vi "LDO Line Transient v2 - Flat.vi"(11 "error in (no error)":errorcluster) -> (15 "error out":errorcluster)   [LabVIEW 2020]
uses:
  <instrlib>/niScope/Controls/niScope vertical coupling.ctl
  <instrlib>/niScope/Controls/niScope trigger source digital.ctl
  <instrlib>/niDCPower/nidcpower.llb/niDCPower Aperture Time Units.ctl
  <instrlib>/niDCPower/nidcpower.llb/niDCPower Source Mode.ctl
  <instrlib>/niDCPower/nidcpower.llb/niDCPower Output Function.ctl
  <instrlib>/niDCPower/nidcpower.llb/niDCPower Export Signal - Signal.ctl
  <instrlib>/niDCPower/nidcpower.llb/niDCPower Wait For Event - Event.ctl
  <instrlib>/niScope/Controls/niScope trigger slope.ctl
  <instrlib>/niScope/Configure/Trigger/niScope Configure Trigger Digital.vi
  <instrlib>/niScope/Acquire/Fetch/niScope Multi Fetch Cluster.vi
  <instrlib>/niScope/Utility/niScope Get Channel Name From String.vi
  <vilib>/gmath/NI_Gmath.lvlib
  LDO Line Transient.lvlib
  <vilib>/gmath/NumericalOptimization/Nonlinear Curve Fit LM formula string.vi
panel:
  out "Horizontal:Number of Records":i32=400000
  out "Horizontal:Min Sample Rate":dbl=1000000.0
  out "Measurement:Measure Record Length":i32=10
  out "Measurement:Aperture Time":dbl=4.9999999999999996e-06
  out "Source:Advanced:Source Delay":dbl=3.086419753086419e-08
  in  "Tab Control":T1(tab)=enum."Waveform"
  in  "Scope":refnum<k15>="PXI1Slot5"
  in  "Load SMU":refnum<k15>="SMU1"
  in  "Source SMU":refnum<k15>="SMU1"
  in  "Load SMU Voltage Limit (V)":dbl=8.0
  in  "Load SMU Voltage Limit Range (V)":dbl=8.0
  in  "Load SMU Current Level Range (A)":dbl=3.0
  in  "Load SMU Channel":string="1"
  in  "Load Current (A)":dbl=-0.05
  in  "Min. Record Length":i32=400000
  in  "Min. Sampling Rate":dbl=1000000.0
  in  "Trigger Modifier":i32(ring) items=["None", "Auto"]
  in  "Reference Position":dbl
  in  "Input Impedance":u32(ring) items=["1 Mega Ohm"=0, "50 Ohm"=2]
  in  "Trigger Delay (sec)":dbl
  in  "Max. Input Frequency (Hz)":dbl
  in  "Vertical Offset (V)":dbl
  in  "Probe Attentuation":dbl=1.0
  in  "Vertical Range (V)":dbl=5.0
  in  "Scope Channel":string="0,1"
  in  "Source SMU Current Limit (A)":dbl=0.2
  in  "Source SMU Transient Response":i32(ring)=1039 items=["Slow"=1041, "Normal"=1038, "Fast"=1039, "Custom"=1042]
  in  "Source SMU Record Length":i32=10
  in  "Source SMU Aperture Time (sec)":dbl=5e-06
  in  "Source SMU Current Limit Range (A)":dbl=0.2
  in  "Source SMU Voltage Level Range (V)":dbl=8.0
  in  "Source SMU Channel":string="0"
  in  "Source  SMU Steady State Voltage (V)":dbl=4.0
  in  "Vertical Coupling":T2 items=["AC", "DC", "Ground"]
  in  "Trigger Source":T3="VAL_PFI_0" caption="trigger source (RTSI 0)"
  in  "Recovery Level (V)":dbl=0.1
  in  "Vin2 Voltage Level Width (sec)":dbl=0.1
  in  "Source Voltage 2 - Vin2":dbl=5.0
  in  "Source Voltage 1 - Vin1":dbl=4.0
  out "Settling time (ms)":dbl=0.008841
  out "Mixed Signal Graph":cluster{waveform(dbl), waveform(dbl)}(graph)={{"t0"=timestamp(0 s since 1904-01-01), "dt"=4.9999999999999996e-06, "Y"=array[40000 elements]}, {"t0"=timestamp(0 s since 1904-01-01), "dt"=4.9999999999999996e-06, "Y"=array[40000 elements]}}
  out "Waveform(s)":T4(graph) caption="Instantaneous Load Transient Waveform"
  out "XY Graph 2":cluster{dbl[], dbl[]}[](graph)
  out "XY Graph":cluster{dbl[], "wfm":dbl[]}[](graph)
  # "Line Transient Measurement - Flat VI"
  # "Source SMU Config"
  # "Scope Config"
  # "Load SMU Config"
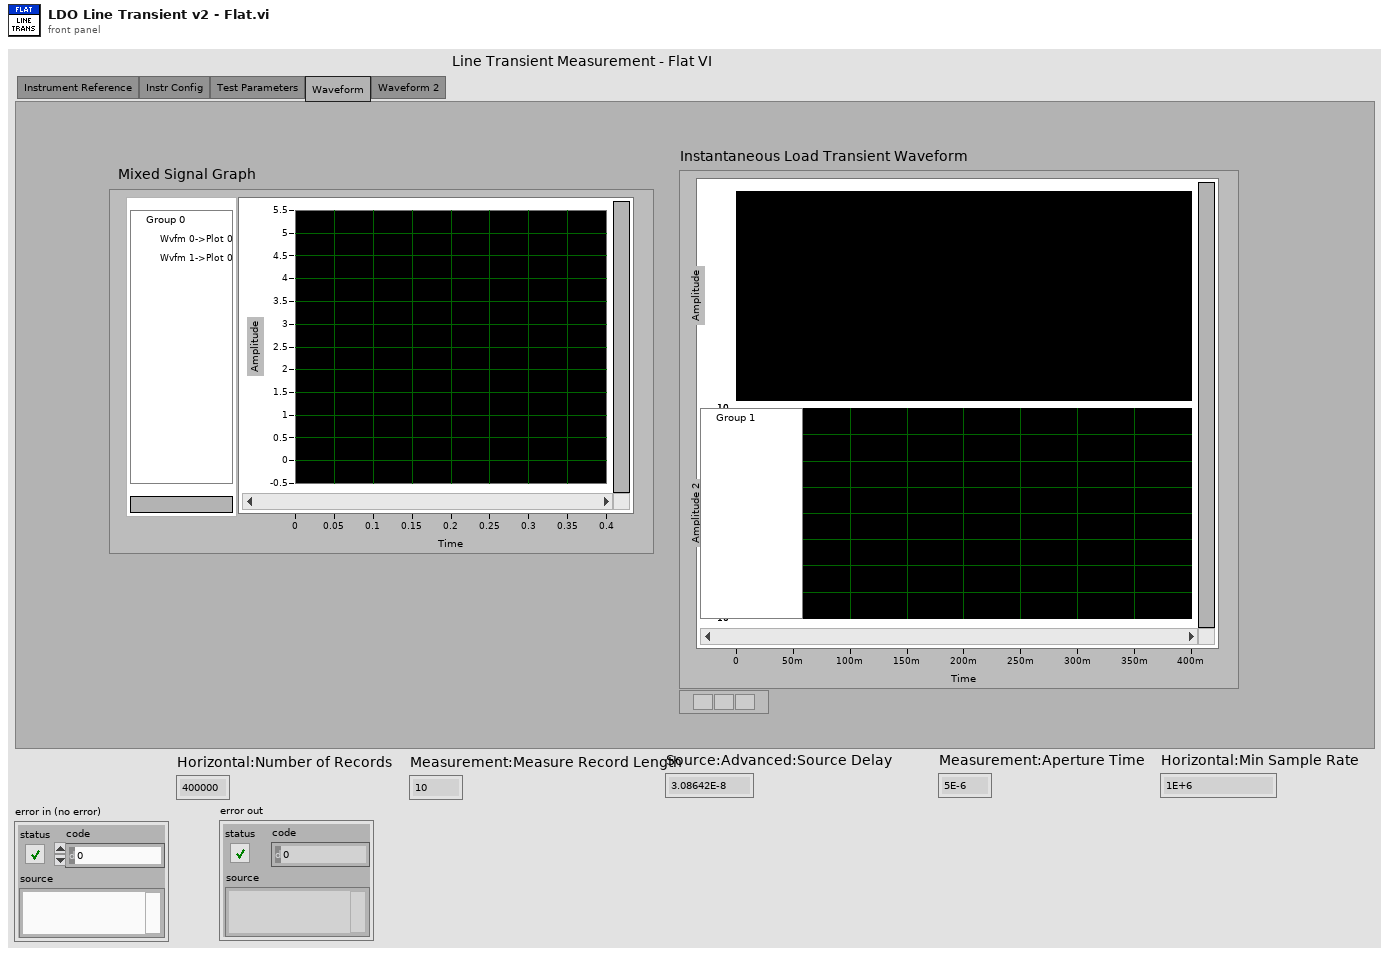
[diagram p1: front panel]
types:
  T1 = enum32{"Instrument Reference", "Instr Config", "Test Parameters", "Waveform", "Waveform 2"}
  T2 = typedef "niScope vertical coupling.ctl" = i32
  T3 = typedef "niScope trigger source digital.ctl" = string
  T4 = cluster{"relativeInitialX":dbl, "xIncrement":dbl, "wfm":dbl[]}[]
  T5 = typedef "niDCPower Output Function.ctl" = i32
  T6 = typedef "niDCPower Source Mode.ctl" = i32
  T7 = typedef "niScope trigger slope.ctl" = i32
  T8 = typedef "niDCPower Wait For Event - Event.ctl" = i32
  T9 = typedef "niDCPower Export Signal - Signal.ctl" = i32
  T10 = typedef "niDCPower Aperture Time Units.ctl" = i32
  T11 = cluster{"relativeInitialX":dbl, "xIncrement":dbl, "wfm":dbl[]}
  T12 = cluster{"model":string, "Parameters":string[], "x":string}
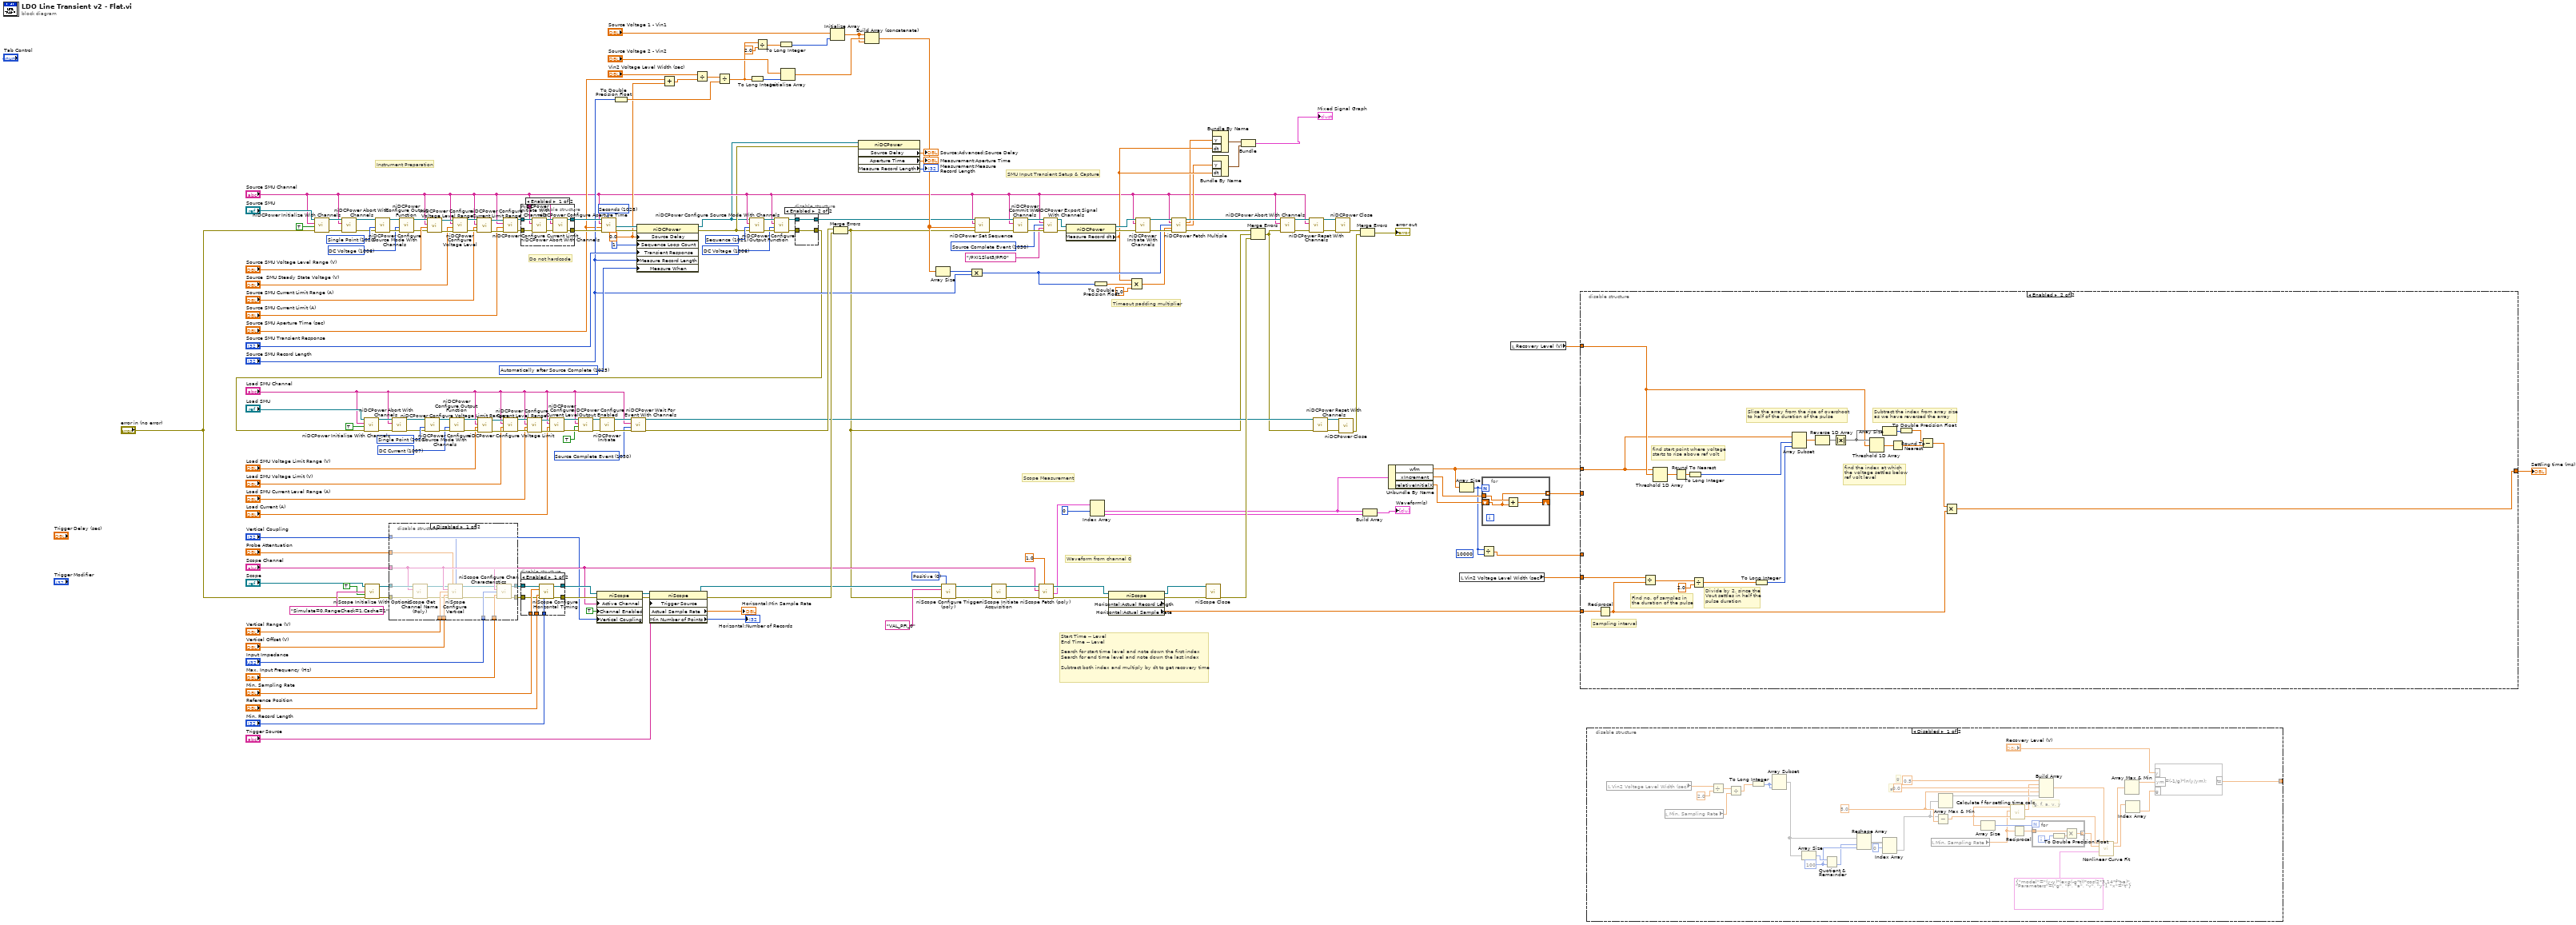
[diagram p0: block diagram]
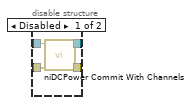
[diagram p4: hidden frame]
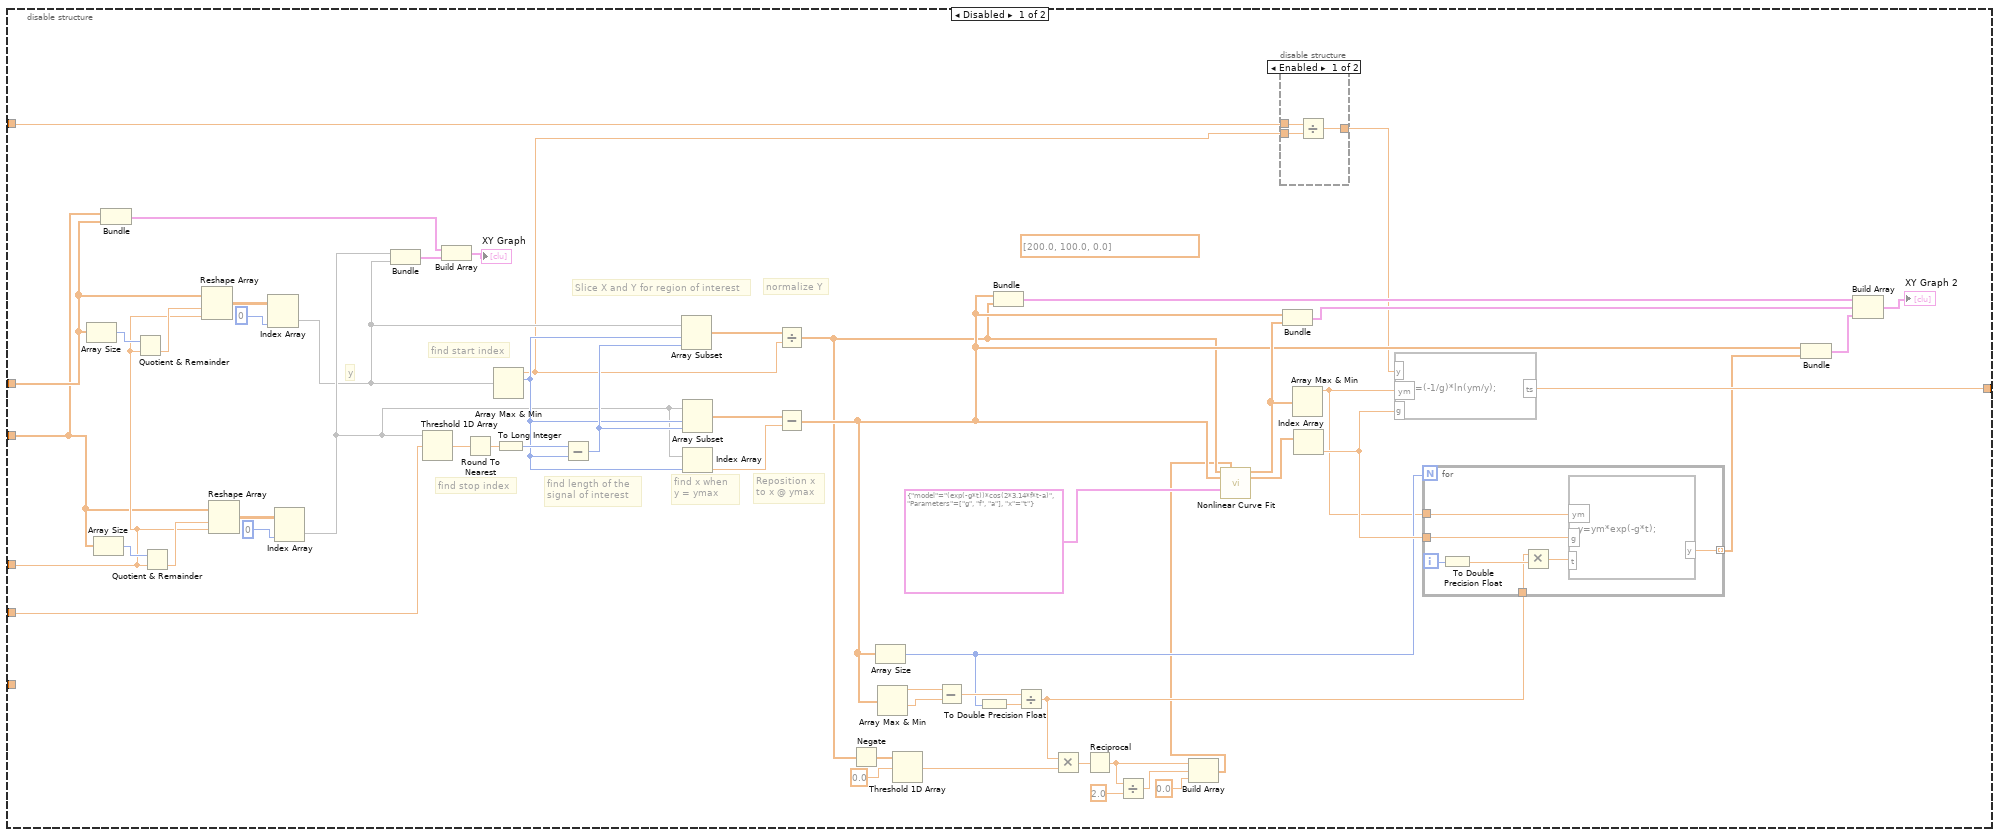
[diagram p5: hidden frame]
diagram:
  (unwired) 10000 ("y")
  w57 = T5 1006 items=["DC Voltage"=1006, "DC Current"=1007, "Pulse Voltage"=1049, "Pulse Current"=1050] ("output function")
  w58 = T6 1021 items=["Single Point"=1020, "Sequence"=1021] ("source mode")
  w51 = T7 0 items=["Positive", "Negative"] ("trigger slope")
  w80 = T8 1030 items=["Source Complete Event"=1030, "Measure Complete Event"=1031, "Sequence Iteration Complete Event"=1032, "Sequence Engine Done Event"=1033, "Pulse Complete Event"=1051, "Ready For Pulse Trigger Event"=1052] ("event")
  w113 = T9 1030 items=["Source Complete Event"=1030, "Measure Complete Event"=1031, "Sequence Iteration Complete Event"=1032, "Sequence Engine Done Event"=1033, "Pulse Complete Event"=1051, "Ready For Pulse Trigger Event"=1052, "Start Trigger"=1034, "Source Trigger"=1035, "Measure Trigger"=1036, "Sequence Advance Trigger"=1037, "Pulse Trigger"=1053] ("signal")
  w153 = T5 1007 items=["DC Voltage"=1006, "DC Current"=1007, "Pulse Voltage"=1049, "Pulse Current"=1050] ("output function")
  w154 = T6 1020 items=["Single Point"=1020, "Sequence"=1021] ("source mode")
  w162 = 1025 items=["Automatically after Source Complete"=1025, "On Demand"=1026, "On Measure Trigger"=1027] ("Measurement:Advanced:Measure When")
  w42 = 0.0 ("Source:Advanced:Source Delay")
  w169 = T10 1028 items=["Seconds"=1028, "Powerline Cycles"=1029] ("aperture time units")
  w172 = T5 1006 items=["DC Voltage"=1006, "DC Current"=1007, "Pulse Voltage"=1049, "Pulse Current"=1050] ("output function")
  w173 = T6 1020 items=["Single Point"=1020, "Sequence"=1021] ("source mode")
  # "Do not hardcode"
  # "Start Time -- Level\nEnd Time -- Level\n\nSearch for start time level and note down the first index\nSearch for end time level and note down the last index\n\nSubtract both index and multiply by dt to get recovery time"
  # "SMU Input Transient Setup & Capture"
  # "Scope Measurement"
  # "Waveform from channel 0"
  # "Timeout padding multiplier"
  # "Instrument Preparation"
  n1 = call <instrlib>:"niDCPower Initialize With Channels.vi"("error in (no error)"="error in (no error)", "reset (false)"=TRUE, "channels"="Source SMU Channel", "resource name"="Source SMU") -> ("error out"=w168:errorcluster, "instrument handle out"=w166:refnum<k15>)  [unwired: 1 in, 5 out]
  n2 = call <instrlib>:"niDCPower Abort With Channels.vi"("error in (no error)"=w168, "channel name"="Source SMU Channel", "instrument handle"=w166) -> ("error out"=w167:errorcluster, "instrument handle out"=w165:refnum<k15>)  [unwired: 7 in]
  n3 = call <instrlib>:"niScope Initialize With Options.vi"("resource name"="Scope", "option string"="Simulate=0,RangeCheck=1,Cache=1", "reset device"=TRUE, "error in"="error in (no error)") -> ("instrument handle"=w139:refnum<k15>, "error out"=w138:errorcluster)  [unwired: 10 in]
  n4 = call <instrlib>:"niDCPower Configure Source Mode With Channels.vi"("error in (no error)"=w167, "source mode"=w173, "instrument handle"=w165) -> ("error out"=w174:errorcluster, "instrument handle out"=w175:refnum<k15>)  [unwired: 7 in]
  n5 = disable-structure shown="Disabled" {
    disable-tunnel: w139 -> [w202 w203]
    disable-tunnel: w138 -> [w201 w204]
    disable-tunnel: "Probe Attentuation" -> [w200 _]
    disable-tunnel: "Vertical Range (V)" -> [w199 _]
    disable-tunnel: "Vertical Offset (V)" -> [w198 _]
    disable-tunnel: "Max. Input Frequency (Hz)" -> [w197 _]
    disable-tunnel: "Input Impedance" -> [w196 _]
    disable-tunnel: "Scope Channel" -> [w195 _]
    disable-tunnel: "Vertical Coupling" -> [w194 _]
    disable-tunnel: [w189 w204] -> w12
    disable-tunnel: [w188 w203] -> w11
    frame Disabled {
      n6 = call-poly <instrlib>:"niScope Get Channel Name (Poly).vi"("instrument handle"=w202, "index"=w195, "error in"=w201) -> ("instrument handle out"=w193:refnum<k15>, "error out"=w192:errorcluster)  [unwired: 10 in, 1 out]
      n7 = call <instrlib>:"niScope Configure Vertical.vi"("instrument handle"=w193, "probe attenuation"=w200, "vertical coupling"=w194, "channels"=w195, "vertical range"=w199, "vertical offset"=w198, "error in"=w192) -> ("instrument handle out"=w191:refnum<k15>, "error out"=w190:errorcluster)  [unwired: 7 in]
      n8 = call <instrlib>:"niScope Configure Chan Characteristics.vi"("instrument handle"=w191, "channels"=w195, "input impedance"=w196, "maximum input frequency"=w197, "error in"=w190) -> ("instrument handle out"=w188:refnum<k15>, "error out"=w189:errorcluster)  [unwired: 9 in]
    }
    frame Enabled {
    }
  }
  n9 = call <instrlib>:"niDCPower Configure Output Function.vi"("error in (no error)"=w174, "output function"=w172, "instrument handle"=w175) -> ("error out"=w170:errorcluster, "instrument handle out"=w171:refnum<k15>)  [unwired: 7 in]
  n10 = call <instrlib>:"niDCPower Configure Voltage Level Range.vi"("error in (no error)"=w170, "voltage level range"="Source SMU Voltage Level Range (V)", "channel name"="Source SMU Channel", "instrument handle"=w171) -> ("error out"=w187:errorcluster, "instrument handle out"=w186:refnum<k15>)  [unwired: 6 in]
  n11 = call <instrlib>:"niDCPower Configure Voltage Level.vi"("error in (no error)"=w187, "voltage level"="Source  SMU Steady State Voltage (V)", "channel name"="Source SMU Channel", "instrument handle"=w186) -> ("error out"=w185:errorcluster, "instrument handle out"=w184:refnum<k15>)  [unwired: 6 in]
  n12 = call <instrlib>:"niDCPower Configure Current Limit Range.vi"("error in (no error)"=w185, "current limit range"="Source SMU Current Limit Range (A)", "channel name"="Source SMU Channel", "instrument handle"=w184) -> ("error out"=w183:errorcluster, "instrument handle out"=w182:refnum<k15>)  [unwired: 6 in]
  n13 = call <instrlib>:"niDCPower Configure Current Limit.vi"("error in (no error)"=w183, "current limit"="Source SMU Current Limit (A)", "channel name"="Source SMU Channel", "instrument handle"=w182) -> ("error out"=w55:errorcluster, "instrument handle out"=w53:refnum<k15>)  [unwired: 6 in]
  n14 = disable-structure shown="Enabled" {
    disable-tunnel: w55 -> [w209 w212]
    disable-tunnel: [w208 w212] -> w54
    disable-tunnel: w53 -> [w207 w213]
    disable-tunnel: [w206 w213] -> w52
    disable-tunnel: "Source SMU Channel" -> [w205 _]
    frame Enabled {
      n15 = call <instrlib>:"niDCPower Initiate With Channels.vi"("error in (no error)"=w209, "channel name"=w205, "instrument handle"=w207) -> ("error out"=w211:errorcluster, "instrument handle out"=w210:refnum<k15>)  [unwired: 7 in]
      n16 = call <instrlib>:"niDCPower Abort With Channels.vi"("error in (no error)"=w211, "channel name"=w205, "instrument handle"=w210) -> ("error out"=w208:errorcluster, "instrument handle out"=w206:refnum<k15>)  [unwired: 7 in]
    }
    frame Disabled {
    }
  }
  n17 = disable-structure shown="Enabled" {
    disable-tunnel: "Min. Record Length" -> [w220 _]
    disable-tunnel: "Reference Position" -> [w219 _]
    disable-tunnel: "Min. Sampling Rate" -> [w218 _]
    disable-tunnel: [w217 w221] -> w21
    disable-tunnel: [w216 w222] -> w19
    disable-tunnel: w12 -> [w215 w221]
    disable-tunnel: w11 -> [w214 w222]
    frame Enabled {
      n18 = call <instrlib>:"niScope Configure Horizontal Timing.vi"("instrument handle"=w214, "min sample rate"=w218, "reference position"=w219, "error in"=w215, "min record length"=w220) -> ("instrument handle out"=w216:refnum<k15>, "error out"=w217:errorcluster)  [unwired: 9 in]
    }
    frame Disabled {
    }
  }
  n19 = property class="niScope"(reference=w19, error in=w21, "Active Channel"="Scope Channel", "Channel Enabled"=TRUE ("Vertical:Channel Enabled"), "Vertical Coupling"="Vertical Coupling") -> (reference out=w18:refnum<k15>, error out=w20:errorcluster)
  n20 = call <instrlib>:"niDCPower Configure Aperture Time.vi"("aperture time units"=w169, "error in (no error)"=w54, "aperture time"="Source SMU Aperture Time (sec)", "channel name"="Source SMU Channel", "instrument handle"=w52) -> ("error out"=w88:errorcluster, "instrument handle out"=w49:refnum<k15>)  [unwired: 5 out]
  n21 = To Double Precision Float(number="Source SMU Record Length") -> (double precision float=w46:dbl)
  n22 = property class="niDCPower"(reference=w49, error in=w88, "Source Delay"=w42, "Sequence Loop Count"=1 ("Source:Advanced:Sequence Loop Count"), "Transient Response"="Source SMU Transient Response", "Measure Record Length"="Source SMU Record Length", "Measure When"=w162) -> (reference out=w22:refnum<k15>, error out=w23:errorcluster)
  n23 = property class="niScope"(reference=w18, error in=w20, "Trigger Source"="Trigger Source") -> (reference out=w75:refnum<k15>, error out=w77:errorcluster, "Actual Sample Rate"=→"Horizontal:Min Sample Rate":dbl, "Min Number of Points"=→"Horizontal:Number of Records":i32)
  n24 = Add(x="Source SMU Aperture Time (sec)", y=w42) -> (x+y=w43:dbl)
  n25 = Divide(x="Vin2 Voltage Level Width (sec)", y=w43) -> (x/y=w48:dbl)
  n26 = Divide(x=w48, y=w46) -> (x/y=w45:dbl)
  n27 = call <instrlib>:"niDCPower Configure Source Mode With Channels.vi"("error in (no error)"=w23, "source mode"=w58, "channel name"="Source SMU Channel", "instrument handle"=w22) -> ("error out"=w59:errorcluster, "instrument handle out"=w56:refnum<k15>)  [unwired: 6 in]
  n28 = To Long Integer(number=w45) -> (32bit integer=w125:i32)
  n29 = Divide(x=w45, y=2.0) -> (x/y=w121:dbl)
  n30 = call <instrlib>:"niDCPower Configure Output Function.vi"("error in (no error)"=w59, "output function"=w57, "channel name"="Source SMU Channel", "instrument handle"=w56) -> ("error out"=w27:errorcluster, "instrument handle out"=w26:refnum<k15>)  [unwired: 6 in]
  n31 = To Long Integer(number=w121) -> (32bit integer=w120:i32)
  n32 = Initialize Array("Source Voltage 2 - Vin2", w125) -> (w119:dbl[])
  n33 = disable-structure shown="Enabled" {
    disable-tunnel: w27 -> [w226 w227]
    disable-tunnel: [w225 w227] -> w9
    disable-tunnel: w26 -> [w224 w228]
    disable-tunnel: [w223 w228] -> w25
    frame Disabled {
      n34 = call <instrlib>:"niDCPower Commit With Channels.vi"("error in (no error)"=w226, "instrument handle"=w224) -> ("error out"=w225:errorcluster, "instrument handle out"=w223:refnum<k15>)  [unwired: 8 in]
    }
    frame Enabled {
    }
  }
  n35 = call <instrlib>:"niDCPower Initialize With Channels.vi"("error in (no error)"=w9, "reset (false)"=TRUE, "channels"="Load SMU Channel", "resource name"="Load SMU") -> ("error out"=w150:errorcluster, "instrument handle out"=w148:refnum<k15>)  [unwired: 1 in, 5 out]
  n36 = call <instrlib>:"niDCPower Abort With Channels.vi"("error in (no error)"=w150, "channel name"="Load SMU Channel", "instrument handle"=w148) -> ("error out"=w149:errorcluster, "instrument handle out"=w147:refnum<k15>)  [unwired: 7 in]
  n37 = call <instrlib>:"niDCPower Configure Source Mode With Channels.vi"("error in (no error)"=w149, "source mode"=w154, "instrument handle"=w147) -> ("error out"=w155:errorcluster, "instrument handle out"=w156:refnum<k15>)  [unwired: 7 in]
  n38 = call <instrlib>:"niDCPower Configure Output Function.vi"("error in (no error)"=w155, "output function"=w153, "instrument handle"=w156) -> ("error out"=w151:errorcluster, "instrument handle out"=w152:refnum<k15>)  [unwired: 7 in]
  n39 = call <instrlib>:"niDCPower Configure Voltage Limit Range.vi"("error in (no error)"=w151, "voltage limit range"="Load SMU Voltage Limit Range (V)", "channel name"="Load SMU Channel", "instrument handle"=w152) -> ("error out"=w161:errorcluster, "instrument handle out"=w160:refnum<k15>)  [unwired: 6 in]
  n40 = call <instrlib>:"niDCPower Configure Voltage Limit.vi"("error in (no error)"=w161, "voltage limit"="Load SMU Voltage Limit (V)", "channel name"="Load SMU Channel", "instrument handle"=w160) -> ("error out"=w159:errorcluster, "instrument handle out"=w158:refnum<k15>)  [unwired: 6 in]
  n41 = call <instrlib>:"niDCPower Configure Current Level Range.vi"("error in (no error)"=w159, "current level range"="Load SMU Current Level Range (A)", "channel name"="Load SMU Channel", "instrument handle"=w158) -> ("error out"=w144:errorcluster, "instrument handle out"=w145:refnum<k15>)  [unwired: 6 in]
  n42 = call <instrlib>:"niDCPower Configure Current Level.vi"("error in (no error)"=w144, "current level"="Load Current (A)", "channel name"="Load SMU Channel", "instrument handle"=w145) -> ("error out"=w85:errorcluster, "instrument handle out"=w82:refnum<k15>)  [unwired: 6 in]
  n43 = call <instrlib>:"niDCPower Configure Output Enabled.vi"("error in (no error)"=w85, "output enabled"=TRUE, "channel name"="Load SMU Channel", "instrument handle"=w82) -> ("error out"=w84:errorcluster, "instrument handle out"=w87:refnum<k15>)  [unwired: 6 in]
  n44 = call <instrlib>:"niDCPower Initiate.vi"("error in (no error)"=w84, "instrument handle"=w87) -> ("error out"=w83:errorcluster, "instrument handle out"=w86:refnum<k15>)  [unwired: 8 in]
  n45 = call <instrlib>:"niDCPower Wait For Event With Channels.vi"("error in (no error)"=w83, "event"=w80, "channel name"="Load SMU Channel", "instrument handle"=w86) -> ("error out"=w78:errorcluster, "instrument handle out"=w63:refnum<k15>)  [unwired: 6 in]
  n46 = Initialize Array("Source Voltage 1 - Vin1", w120) -> (w118:dbl[])
  n47 = Merge Errors(w78, w77) -> (w7:errorcluster)
  n48 = property class="niDCPower"(reference=w22, error in=w23) -> ("Source Delay"=→"Source:Advanced:Source Delay":dbl, "Aperture Time"=→"Measurement:Aperture Time":dbl, "Measure Record Length"=→"Measurement:Measure Record Length":i32)  [unwired: 2 out]
  n49 = Build Array (concatenate)(w118, w119, w118) -> (w109:dbl[])
  n50 = Array Size(array=w109) -> (size(s)=w108:i32)
  n51 = call-poly <instrlib>:"niScope Configure Trigger (poly).vi"("instrument handle"=w75, "trigger slope"=w51, "trigger source"=T3 "VAL_PFI_0", "error in"=w7) -> ("instrument handle out"=w76:refnum<k15>, "error out"=w90:errorcluster)  [unwired: 10 in]
  n52 = Compound Arithmetic op=MULTIPLY(w108, "Source SMU Record Length") -> (w101:i32)
  n53 = call <instrlib>:"niDCPower Set Sequence.vi"("error in (no error)"=w7, "values"=w109, "channel name"="Source SMU Channel", "instrument handle"=w25) -> ("error out"=w117:errorcluster, "instrument handle out"=w116:refnum<k15>)  [unwired: 1 in, 5 out]
  n54 = call <instrlib>:"niScope Initiate Acquisition.vi"("instrument handle"=w76, "error in"=w90) -> ("instrument handle out"=w73:refnum<k15>, "error out"=w89:errorcluster)  [unwired: 12 in]
  n55 = call <instrlib>:"niDCPower Commit With Channels.vi"("error in (no error)"=w117, "channel name"="Source SMU Channel", "instrument handle"=w116) -> ("error out"=w115:errorcluster, "instrument handle out"=w114:refnum<k15>)  [unwired: 7 in]
  n56 = call-poly <instrlib>:"niScope Fetch (poly).vi"("timeout"=1.0, "error in"=w89, "channels"="Scope Channel", "instrument handle"=w73) -> ("error out"=w91:errorcluster, "waveform"=w70:T4, "instrument handle out"=w71:refnum<k15>)  [unwired: 4 in, 1 out]
  n57 = call <instrlib>:"niDCPower Export Signal With Channels.vi"("instrument handle"=w114, "channel name"="Source SMU Channel", "signal"=w113, "output terminal"=tag "/PXI1Slot5/PFI0", "error in (no error)"=w115) -> ("instrument handle out"=w110:refnum<k15>, "error out"=w111:errorcluster)  [unwired: 9 in]
  n58 = property class="niDCPower"(reference=w110, error in=w111) -> (reference out=w104:refnum<k15>, error out=w105:errorcluster, "Measure Record dt"=w94:dbl)
  n59 = Index Array(array=w70, index #1=0 ("index")) -> (element #1=w41:T11, element #2=w1:T11)  [unwired: 1 in]
  n60 = To Double Precision Float(number=w101) -> (double precision float=w106:dbl)
  n61 = property class="niScope" props=["Horizontal:Actual Record Length", "Horizontal:Actual Sample Rate"](reference=w71, error in=w91) -> (reference out=w67:refnum<k15>, error out=w68:errorcluster, "Horizontal:Actual Sample Rate"=w31:dbl)  [unwired: 1 out]
  n62 = Compound Arithmetic op=MULTIPLY(w94, w106, 2.0 ("value")) -> (w100:dbl)
  n63 = call <instrlib>:"niDCPower Initiate With Channels.vi"("error in (no error)"=w105, "channel name"="Source SMU Channel", "instrument handle"=w104) -> ("error out"=w103:errorcluster, "instrument handle out"=w102:refnum<k15>)  [unwired: 7 in]
  n64 = call <instrlib>:"niDCPower Fetch Multiple.vi"("instrument handle"=w102, "channel name"="Source SMU Channel", "count (1)"=w101, "timeout (sec)"=w100, "error in (no error)"=w103) -> ("instrument handle out"=w99:refnum<k15>, "voltage measurements"=w62:dbl[], "current measurements"=w93:dbl[], "error out"=w8:errorcluster)  [unwired: 7 out]
  n65 = call <instrlib>:"niScope Close.vi"("instrument handle"=w67, "error in"=w68) -> ("error out"=w66:errorcluster)  [unwired: 13 in]
  n66 = Bundle By Name("Y"=w62, "dt"=w94) -> (w92:waveform(dbl))  [unwired: 1 out]
  n67 = Bundle By Name("Y"=w93, "dt"=w94) -> (w61:waveform(dbl))  [unwired: 1 out]
  n68 = Bundle(w92, w61) -> (→"Mixed Signal Graph":cluster{waveform(dbl), waveform(dbl)})  [unwired: 1 in]
  n69 = Merge Errors(w8, w7, w66) -> (w6:errorcluster)
  n70 = call <instrlib>:"niDCPower Abort With Channels.vi"("error in (no error)"=w6, "channel name"="Source SMU Channel", "instrument handle"=w99) -> ("error out"=w97:errorcluster, "instrument handle out"=w95:refnum<k15>)  [unwired: 7 in]
  n71 = call <instrlib>:"niDCPower Reset With Channels.vi"("error in (no error)"=w97, "channel name"="Source SMU Channel", "instrument handle"=w95) -> ("error out"=w96:errorcluster, "instrument handle out"=w98:refnum<k15>)  [unwired: 7 in]
  n72 = call <instrlib>:"niDCPower Reset With Channels.vi"("error in (no error)"=w6, "instrument handle"=w63) -> ("error out"=w64:errorcluster, "instrument handle out"=w65:refnum<k15>)  [unwired: 8 in]
  n73 = call <instrlib>:"niDCPower Close.vi"("error in (no error)"=w96, "instrument handle"=w98) -> ("error out"=w5:errorcluster)  [unwired: 9 out]
  n74 = call <instrlib>:"niDCPower Close.vi"("error in (no error)"=w64, "instrument handle"=w65) -> ("error out"=w4:errorcluster)  [unwired: 9 out]
  n75 = Merge Errors(w5, w4) -> (→"error out":errorcluster)
  n76 = Build Array(w41, w1) -> (→"Waveform(s)":T4)
  n77 = Unbundle By Name(w41) -> ("wfm"=w36:dbl[], "xIncrement"=w39:dbl, "relativeInitialX"=w40:dbl)
  n78 = Array Size(array=w36) -> (size(s)=w34:i32)
  n79 = local read "Vin2 Voltage Level Width (sec)"() -> (w33:dbl)
  n80 = Divide(x=w34, y=w34) -> (x/y=w37:dbl)
  n81 = for {
    N: w34 -> [_]
    tunnel: w39 -> [w231]
    shift-right: [w230] -> _
    shift-left: w40 -> [w229]
    tunnel: [w229] -> w35 mode=indexing
    n82 = Add(x=w231, y=w229) -> (x+y=w230:dbl)
  }
  n83 = local read "Recovery Level (V)"() -> (w32:dbl)
  n84 = disable-structure shown="Enabled" {
    disable-tunnel: [w277 w303] -> w38
    disable-tunnel: w37 -> [w258 _]
    disable-tunnel: w36 -> [w241 w300]
    disable-tunnel: w35 -> [w240 _]
    disable-tunnel: w33 -> [w233 w299]
    disable-tunnel: w32 -> [w232 w301]
    disable-tunnel: w31 -> [_ w302]
    frame Disabled {
      (unwired) dbl[] [200.0, 100.0, 0.0] ("initial parameters")
      # "find x when \ny = ymax"
      # "Reposition x \nto x @ ymax"
      # "normalize Y"
      # "Slice X and Y for region of interest"
      # "find length of the \nsignal of interest"
      # "find stop index"
      # "find start index"
      # "y"
      n85 = Array Size(array=w241) -> (size(s)=w267:i32)
      n86 = Array Size(array=w240) -> (size(s)=w271:i32)
      n87 = Bundle(w240, "wfm"=w241) -> (w238:cluster{dbl[], "wfm":dbl[]})  [unwired: 1 in]
      n88 = Quotient & Remainder(x=w267, y=w258) -> (floor(x/y)=w266:dbl)  [unwired: 1 out]
      n89 = Quotient & Remainder(x=w271, y=w258) -> (floor(x/y)=w270:dbl)  [unwired: 1 out]
      n90 = Reshape Array(w241, w266, w258) -> (w265:dbl[][])
      n91 = Reshape Array(w240, w270, w258) -> (w269:dbl[][])
      n92 = Index Array(array=w265, index (col)=0 ("index (row)")) -> (element=w264:dbl[])  [unwired: 1 in]
      n93 = Index Array(array=w269, index (col)=0 ("index (row)")) -> (element=w268:dbl[])  [unwired: 1 in]
      n94 = Bundle(w268, "wfm"=w264) -> (w275:cluster{dbl[], "wfm":dbl[]})  [unwired: 1 in]
      n95 = Threshold 1D Array(2:w233, 3:w268) -> (0:w286:dbl)  [unwired: 1 in]
      n96 = Build Array(w238, w275) -> (→"XY Graph":cluster{dbl[], "wfm":dbl[]}[])
      n97 = Round To Nearest(number=w286) -> (nearest integer value=w287:dbl)
      n98 = Array Max & Min(array=w264) -> (max value=w236:dbl, max index (indices)=w281:i32)  [unwired: 2 out]
      n99 = To Long Integer(number=w287) -> (32bit integer=w285:i32)
      n100 = Subtract(x=w285, y=w281) -> (x-y=w284:i32)
      n101 = Array Subset(array=w264, index=w281, length=w284) -> (w283:dbl[])
      n102 = Array Subset(array=w268, index=w281, length=w284) -> (w282:dbl[])
      n103 = Index Array(array=w268, index=w281) -> (element=w280:dbl)
      n104 = Divide(x=w283, y=w236) -> (x/y=w251:dbl[])
      n105 = Subtract(x=w282, y=w280) -> (x-y=w257:dbl[])
      n106 = Negate(x=w251) -> (-x=w250:dbl[])
      n107 = Array Size(array=w257) -> (size(s)=w253:i32)
      n108 = Array Max & Min(array=w257) -> (max value=w256:dbl, min value=w255:dbl)  [unwired: 2 out]
      n109 = Threshold 1D Array(2:0.0 ("threshold y"), 3:w250) -> (0:w248:dbl)  [unwired: 1 in]
      n110 = Subtract(x=w256, y=w255) -> (x-y=w254:dbl)
      n111 = To Double Precision Float(number=w253) -> (double precision float=w252:dbl)
      n112 = Bundle(w257, w251) -> (w276:cluster{dbl[], dbl[]})  [unwired: 1 in]
      n113 = Divide(x=w254, y=w252) -> (x/y=w247:dbl)
      n114 = Multiply(x=w247, y=w248) -> (x*y=w246:dbl)
      n115 = Reciprocal(x=w246) -> (1/x=w245:dbl)
      n116 = Divide(x=w245, y=2.0) -> (x/y=w243:dbl)
      n117 = Build Array(w245, w243, 0.0 ("element")) -> (w234:dbl[])
      n118 = call-poly <vilib>:"Nonlinear Curve Fit.vi"("Y"=w251, "initial parameters"=w234, "X"=w257, "model description"=T12 {"model"="(exp(-g*t))*cos(2*3.14*f*t-a)", "Parameters"=["g", "f", "a"], "x"="t"}) -> ("best nonlinear fit"=w274:dbl[], "best fit parameters"=w278:dbl[])  [unwired: 7 in, 3 out]
      n119 = disable-structure shown="Enabled" {
        disable-tunnel: w232 -> [w290 w291]
        disable-tunnel: [w289 w291] -> w237
        disable-tunnel: w236 -> [w288 _]
        frame Enabled {
          n120 = Divide(x=w290, y=w288) -> (x/y=w289:dbl)
        }
        frame Disabled {
        }
      }
      n121 = Bundle(w257, "best nonlinear fit"=w274) -> (w272:cluster{dbl[], "best nonlinear fit":dbl[]})  [unwired: 1 in]
      n122 = Array Max & Min(array=w274) -> (max value=w235:dbl)  [unwired: 3 out]
      n123 = Index Array(array=w278) -> (element=w261:dbl)  [unwired: 1 in]
      n124 = formula code="ts =(-1/g)*ln(ym/y);"("y"=w237, "ym"=w235, "g"=w261) -> ("ts"=w277:dbl)
      n125 = for {
        N: w253 -> [_]
        tunnel: [w297] -> w260 mode=indexing
        tunnel: w261 -> [w294]
        tunnel: w235 -> [w293]
        tunnel: w247 -> [w292]
        i -> [w298]
        n126 = To Double Precision Float(number=w298) -> (double precision float=w295:dbl)
        n127 = Multiply(x=w292, y=w295) -> (x*y=w296:dbl)
        n128 = formula code="y=ym*exp(-g*t);"("g"=w294, "ym"=w293, "t"=w296) -> ("y"=w297:dbl)
      }
      n129 = Bundle(w257, w260) -> (w259:cluster{dbl[], dbl[]})  [unwired: 1 in]
      n130 = Build Array(w276, w272, w259) -> (→"XY Graph 2":cluster{dbl[], "best nonlinear fit":dbl[]}[])
    }
    frame Enabled {
      # "Subtract the index from array size\nas we have reversed the array"
      # "Sampling interval"
      # "find the index at which \nthe voltage settles below\nref volt level"
      # "Slice the array from the rise of overshoot\nto half of the duration of the pulse"
      # "Divide by 2, since the\nVout settles in half the\npulse duration"
      # "Find no. of samples in \nthe duration of the pulse"
      # "find start point where voltage\nstarts to rise above ref volt"
      n131 = Reciprocal(x=w302) -> (1/x=w311:dbl)
      n132 = Divide(x=w299, y=w311) -> (x/y=w317:dbl)
      n133 = Threshold 1D Array(2:w301, 3:w300) -> (0:w319:dbl)  [unwired: 1 in]
      n134 = Round To Nearest(number=w319) -> (nearest integer value=w318:dbl)
      n135 = To Long Integer(number=w318) -> (32bit integer=w310:i32)
      n136 = Divide(x=w317, y=2.0) -> (x/y=w315:dbl)
      n137 = To Long Integer(number=w315) -> (32bit integer=w314:i32)
      n138 = Array Subset(array=w300, index=w310, length=w314) -> (w309:dbl[])
      n139 = Reverse 1D Array(array=w309) -> (reversed array=w313:dbl[])
      n140 = Absolute Value(x=w313) -> (abs(x)=w306:dbl[])
      n141 = Threshold 1D Array(2:w301, 3:w306) -> (0:w312:dbl)  [unwired: 1 in]
      n142 = Array Size(array=w306) -> (size(s)=w305:i32)
      n143 = Round To Nearest(number=w312) -> (nearest integer value=w308:dbl)
      n144 = To Double Precision Float(number=w305) -> (double precision float=w304:dbl)
      n145 = Subtract(x=w304, y=w308) -> (x-y=w307:dbl)
      n146 = Multiply(x=w307, y=w311) -> (x*y=w303:dbl)
    }
  }
  "Settling time (ms)" <- w38
  n147 = disable-structure shown="Disabled" {
    disable-tunnel: [w320 _] -> _
    frame Disabled {
      w326 = 100 ("y")
      w330 = 5.0 ("element")
      # "a"
      # "g"
      # "g, f, a, v, y"
      n148 = local read "Vin2 Voltage Level Width (sec)"() -> (w346:dbl)
      n149 = local read "Min. Sampling Rate"() -> (w328:dbl)
      n150 = Divide(x=w346, y=2.0) -> (x/y=w349:dbl)
      n151 = Divide(x=w349, y=w328) -> (x/y=w348:dbl)
      n152 = To Long Integer(number=w348) -> (32bit integer=w347:i32)
      n153 = Array Subset(index=w347, length=w347) -> (w322:void[])  [unwired: 1 in]
      n154 = Array Size(array=w322) -> (size(s)=w327:i32)
      n155 = Quotient & Remainder(x=w327, y=w326) -> (floor(x/y)=w325:i32)  [unwired: 1 out]
      n156 = Reshape Array(w322, w325, w326) -> (w324:void[][])
      n157 = Index Array(array=w324, index (row)=0) -> (element=w321:void[])  [unwired: 1 in]
      n158 = local read "Min. Sampling Rate"() -> (w331:dbl)
      n159 = Subtract(x=w321, y=w330) -> (x-y=w339:dbl)
      n160 = Array Max & Min(array=w321) -> (max value=w341)  [unwired: 3 out]
      n161 = Array Size(array=w339) -> (size(s)=w342:i32)
      n162 = call "Calculate f for settling time calc.vi"("Sampling Freq (Hz)"=w331, "Scope Waveform"=w339) -> ("Frequency 'f'"=w338:dbl)  [unwired: 3 in]
      n163 = Reciprocal(x=w331) -> (1/x=w344:dbl)
      n164 = for {
        N: w342 -> [_]
        tunnel: w344 -> [w354]
        tunnel: [w351] -> w343 mode=indexing
        i -> [w353]
        n165 = To Double Precision Float(number=w353) -> (double precision float=w352:dbl)
        n166 = Multiply(x=w354, y=w352) -> (x*y=w351:dbl)
      }
      n167 = Build Array(0.5 ("element"), w338, 0.0 ("element"), w330, w341) -> (w336:dbl[])
      n168 = call-poly <vilib>:"Nonlinear Curve Fit.vi"("Y"=w339, "initial parameters"=w336, "X"=w343, "model description"=T12 {"model"="(y-v)*(exp(-g*t))*cos(2*3.14*f*t-a)", "Parameters"=["g", "f", "a", "v", "y"], "x"="t"}) -> ("best nonlinear fit"=w335:dbl[], "best fit parameters"=w334:dbl[])  [unwired: 7 in, 3 out]
      n169 = Array Max & Min(array=w335) -> (max value=w333:dbl)  [unwired: 3 out]
      n170 = Index Array(array=w334) -> (element=w332:dbl)  [unwired: 1 in]
      n171 = formula code="ts =(-1/g)*ln(y/ym);"("y"="Recovery Level (V)", "ym"=w333, "g"=w332) -> ("ts"=w320:dbl)
    }
    frame Enabled {
    }
  }
